vi "6.3.DHT22 Temp-Humidity Sensor -ThingSpeak-SDCard.vi"   [LabVIEW 2014]
uses:
  <vilib>/Aledyne-TSXperts/Arduino Compatible Compiler for LabVIEW/addons/QwaveSys_ESP8266/QwaveSys_ESP8266.lvlib
  <vilib>/Aledyne-TSXperts/Arduino Compatible Compiler for LabVIEW/addons/QwaveSys_Interface/QwaveSys_Interface.lvlib
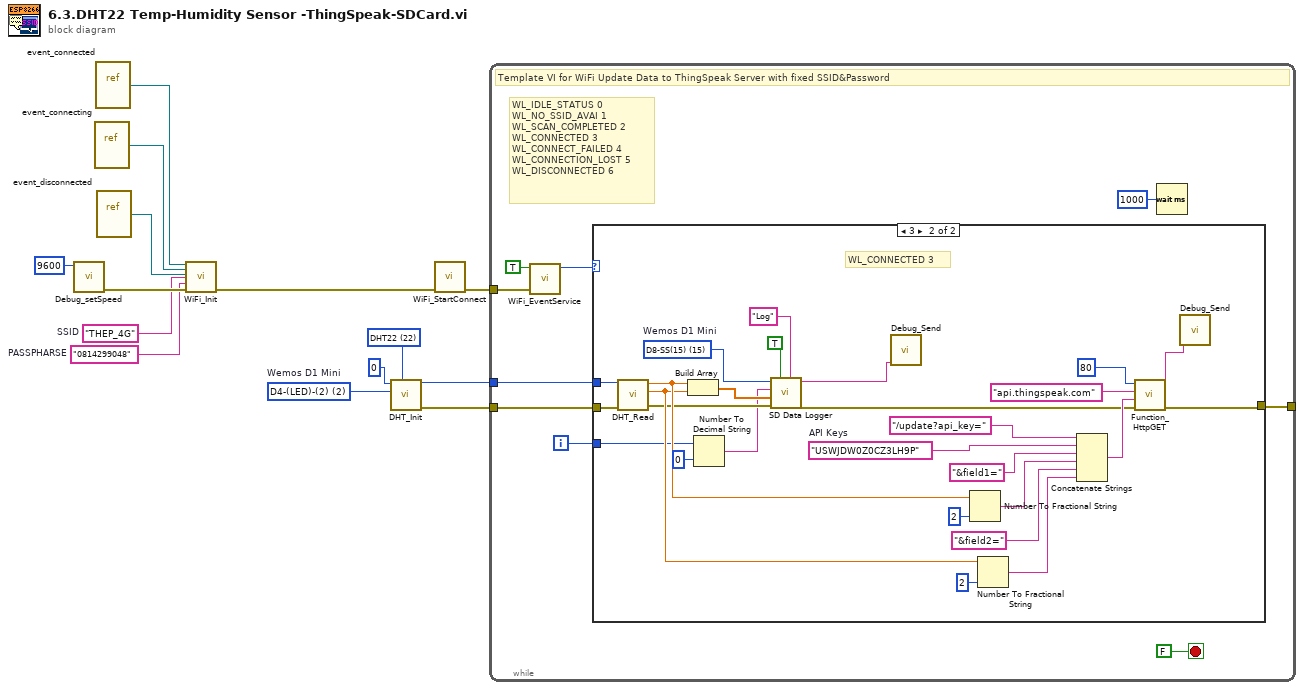
[diagram p0: block diagram]
diagram:
  w3 = u8 2 items=["D0-(16)"=16, "D1-SCL(5)"=5, "D2-SDA(4)"=4, "D3-(0)"=0, "D4-(LED)-(2)"=2, "D5-SCK(14)"=14, "D6-MISO(12)"=12, "D7-MOSI(13)"=13, "D8-SS(15)"=15, "TX(3)"=3, "RX(1)"=1, "ADC0,(17)"=17]  # Wemos D1 Mini
  w5 = u16 22 items=["DHT11"=11, "DHT21"=21, "DHT22"=22] ("Type")
  w7 = "0814299048"  # PASSPHARSE
  w8 = "THEP_4G"  # SSID
  n1 = call <vilib>:"Debug_setSpeed.vi"("Speed"=u32 9600) -> ("error out"=w10:errorcluster)  [unwired: 10 in]
  n2 = vi-ref "event_connecting.vi"() -> (w13:refnum<vi>)
  n3 = vi-ref "event_connected.vi"() -> (w12:refnum<vi>)
  n4 = vi-ref "event_disconnected.vi"() -> (w11:refnum<vi>)
  n5 = call <vilib>:"WiFi_Init.vi"("connected"=w12, "connecting"=w13, "disconnected"=w11, "SSID"=w8, "PASSPHARSE"=w7, "error in (no error)"=w10) -> ("error out"=w6:errorcluster)  [unwired: 9 in]
  n6 = call <vilib>:"DHT_Init.vi"("Type"=w5, "PIN"=w3, "Interface (0-4)"=u8 0) -> ("error out"=w2:errorcluster, "Instance"=w1:u8)  [unwired: 7 in]
  n7 = call <vilib>:"WiFi_StartConnect.vi"("error in (no error)"=w6) -> ("error out"=w14:errorcluster)  [unwired: 10 in]
  n8 = while {
    tunnel: w14 -> [w22]
    tunnel: [w18] -> _
    tunnel: w2 -> [w17]
    tunnel: w1 -> [w16]
    i -> [w15]
    stop <- FALSE stop-if-true
    # "WL_IDLE_STATUS\t0\nWL_NO_SSID_AVAI\t1\nWL_SCAN_COMPLETED\t2\nWL_CONNECTED\t3\nWL_CONNECT_FAILED\t4\nWL_CONNECTION_LOST\t5\nWL_DISCONNECTED\t6"
    # "Template VI for WiFi Update Data to ThingSpeak Server with fixed SSID&Password"
    n9 = call <vilib>:"WiFi_EventService.vi"("error in (no error)"=w22, "wait for connected (True)"=TRUE) -> ("Status"=w19:u16)  [unwired: 8 in, 1 out]
    n10 = case shown="3" w19 {
      tunnel: [w24 w37] -> w18
      tunnel: w17 -> [w24 w39]
      tunnel: w16 -> [_ w38]
      tunnel: w15 -> [_ w28]
      frame 0, Default {
        # "DISCONNECTED or default status"
      }
      frame 3 {
        w29 = u8 15 items=["D0-(16)"=16, "D1-SCL(5)"=5, "D2-SDA(4)"=4, "D3-(0)"=0, "D4-(LED)-(2)"=2, "D5-SCK(14)"=14, "D6-MISO(12)"=12, "D7-MOSI(13)"=13, "D8-SS(15)"=15, "TX(3)"=3, "RX(1)"=1, "ADC0,(17)"=17]  # Wemos D1 Mini
        w42 = "USWJDW0Z0CZ3LH9P"  # API Keys
        # "WL_CONNECTED\t3"
        n11 = call <vilib>:"DHT_Read.vi"("Instance"=w38, "error in (no error)"=w39) -> ("error out"=w34:errorcluster, "Celsius"=w35:dbl, "Humidity"=w36:dbl)  [unwired: 4 in, 3 out]
        n12 = Build Array(w36, w35) -> (w30:dbl[])
        n13 = Number To Decimal String(number=w28, width (-)=i16 0) -> (decimal integer string=w27:string)
        n14 = call <vilib>:"SD Data Logger.vi"("File Name"="Log", "Append Timestamp"=TRUE, "error in (no error)"=w34, "Data"=w30, "Timestamp"=w27, "CS Pin"=w29) -> ("error out"=w33:errorcluster, "CSV Data"=w26:string)  [unwired: 4 in]
        n15 = call <vilib>:"Debug_Send.vi"("DATA"=w26) -> ()  [unwired: 11 in]
        n16 = Number To Fractional String(number=w36, precision (6)=i16 2) -> (F-format string=w46:string)  [unwired: 2 in]
        n17 = Number To Fractional String(number=w35, precision (6)=i16 2) -> (F-format string=w49:string)  [unwired: 2 in]
        n18 = Concatenate Strings("/update?api_key=", w42, "&field1=", w46, "&field2=", w49) -> (w43:string)
        n19 = call <vilib>:"Function_HttpGET.vi"("error in (no error)"=w33, "URI"=w43, "Host"="api.thingspeak.com", "Port"=i8 80) -> ("error out"=w37:errorcluster, "Results"=w40:string)  [unwired: 6 in]
        n20 = call <vilib>:"Debug_Send.vi"("DATA"=w40) -> ()  [unwired: 11 in]
      }
    }
    n21 = Wait (ms)(milliseconds to wait=u32 1000) -> ()  [unwired: 1 out]
  }
